vi "test_methods.vi"() -> ()   [LabVIEW 2021]
uses:
  Parent/Parent.lvclass
  Child/Child.lvclass
panel:
  out "message 6":string="Parent Dynamic VI"
  out "message 5":string="Parent Static  VI"
  out "message 4":string="Parent Static  VI"
  out "message 3":string="Child Dynamic VI"
  out "message 2":string="Parent Dynamic VI"
  out "message 1":string="Parent Static  VI"
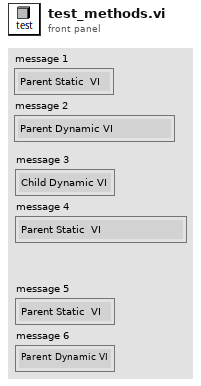
[diagram p1: front panel]
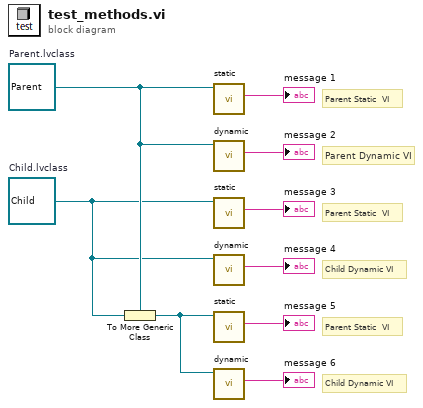
[diagram p0: block diagram]
diagram:
  w6 = refnum<class "Child.lvclass"> refnum  # Child.lvclass
  w7 = refnum<class "Parent.lvclass"> refnum  # Parent.lvclass
  # "Child Dynamic VI"
  # "Child Dynamic VI"
  # "Parent Dynamic VI"
  # "Parent Static  VI"
  # "Parent Static  VI"
  # "Parent Static  VI"
  n1 = To More Generic Class(target class=w7, reference=w6) -> (generic class reference=w3:refnum<class "Parent.lvclass">)
  n2 = call "static.vi"("parent in"=w7) -> ("message"=→"message 1":string)  [unwired: 8 in, 2 out]
  n3 = call-dynamic "dynamic.vi"("parent in"=w7) -> ("message"=→"message 2":string)  [unwired: 8 in, 2 out]
  n4 = call "static.vi"("parent in"=w6) -> ("message"=→"message 3":string)  [unwired: 8 in, 2 out]
  n5 = call-dynamic "dynamic.vi"("Child in"=w6) -> ("message"=→"message 4":string)  [unwired: 8 in, 2 out]
  n6 = call "static.vi"("parent in"=w3) -> ("message"=→"message 5":string)  [unwired: 8 in, 2 out]
  n7 = call-dynamic "dynamic.vi"("parent in"=w3) -> ("message"=→"message 6":string)  [unwired: 8 in, 2 out]
